vi "TrigerDelayer_ABCDEFGHDelay_Set.vi"(8 "error in (no error)":errorcluster, 10 "ABCDEFGH Delay(ns)":T1, 11 "VISA Refnum in":refnum<visa-resource-name>) -> (0 "error out":errorcluster, 3 "VISA Refnum out":refnum<visa-resource-name>)   [LabVIEW 2016, in "Trigger Delayer.lvlib"]
doc: "设置延时器的各个延时，用于同步。"
uses:
  TrigerDelayer_ABCDEFGHDelay_ctl.ctl
  Trigger Delayer.lvlib
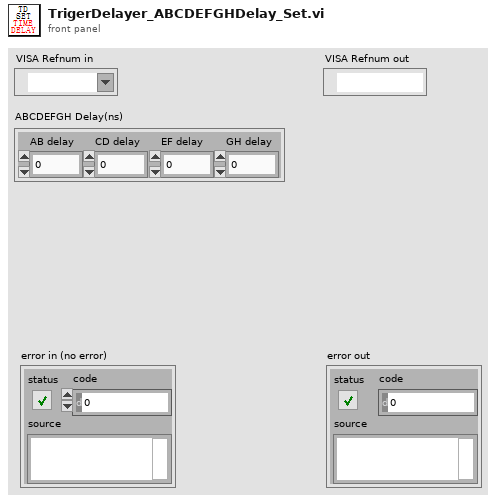
[diagram p1: front panel]
types:
  T1 = typedef "Trigger Delayer.lvlib/TrigerDelayer_ABCDEFGHDelay_ctl.ctl" = cluster{"AB delay":dbl, "CD delay":dbl, "EF delay":dbl, "GH delay":dbl}
  T2 = cluster{"AB delay":dbl, "CD delay":dbl, "EF delay":dbl, "GH delay":dbl}
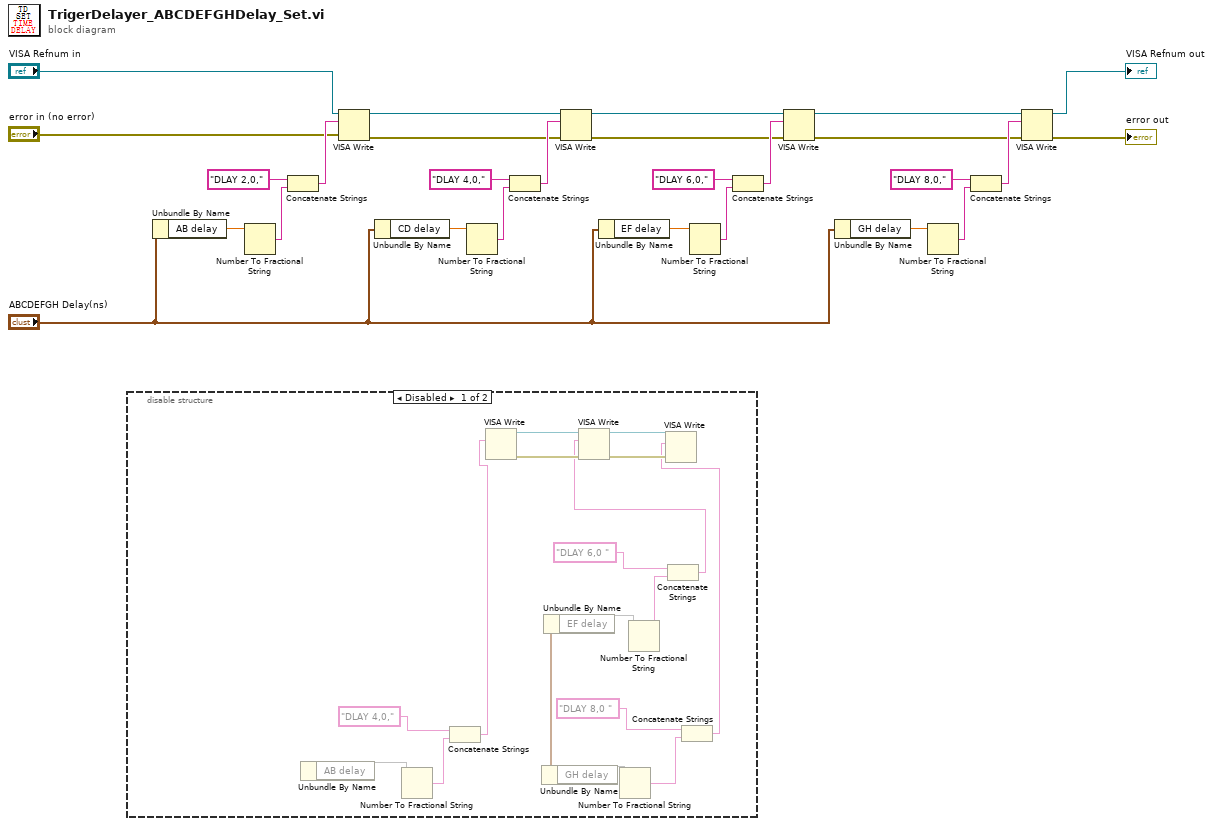
[diagram p0: block diagram]
diagram:
  n1 = disable-structure shown="Disabled" {
    frame Disabled {
      n2 = Unbundle By Name() -> (w28:T2, "AB delay"=w32)
      n3 = Number To Fractional String(number=w32) -> (F-format string=w33:string)  [unwired: 3 in]
      n4 = Concatenate Strings("DLAY 4,0,", w33) -> (w39:string)
      n5 = VISA Write(write buffer=w39) -> (VISA resource name=w42:refnum<visa-resource-name>, error in (no error)=w43:errorcluster, VISA resource name out=w44:refnum<visa-resource-name>, error out=w45:errorcluster)  [unwired: 1 out]
      n6 = Unbundle By Name() -> (w29:T2, "EF delay"=w31)
      n7 = Unbundle By Name(w29) -> ("GH delay"=w30)
      n8 = Number To Fractional String(number=w30) -> (F-format string=w38:string)  [unwired: 3 in]
      n9 = Number To Fractional String(number=w31) -> (F-format string=w35:string)  [unwired: 3 in]
      n10 = Concatenate Strings("DLAY 6,0 ", w35) -> (w40:string)
      n11 = VISA Write(VISA resource name=w44, write buffer=w40, error in (no error)=w45) -> (VISA resource name out=w46:refnum<visa-resource-name>, error out=w47:errorcluster)  [unwired: 1 out]
      n12 = Concatenate Strings("DLAY 8,0 ", w38) -> (w41:string)
      n13 = VISA Write(VISA resource name=w46, write buffer=w41, error in (no error)=w47) -> ()  [unwired: 3 out]
    }
    frame Enabled {
    }
  }
  n14 = Unbundle By Name("ABCDEFGH Delay(ns)") -> ("AB delay"=w22:dbl)
  n15 = Number To Fractional String(number=w22) -> (F-format string=w25:string)  [unwired: 3 in]
  n16 = Concatenate Strings("DLAY 2,0,", w25) -> (w27:string)
  n17 = VISA Write(VISA resource name="VISA Refnum in", write buffer=w27, error in (no error)="error in (no error)") -> (VISA resource name out=w9:refnum<visa-resource-name>, error out=w8:errorcluster)  [unwired: 1 out]
  n18 = Unbundle By Name("ABCDEFGH Delay(ns)") -> ("CD delay"=w21:dbl)
  n19 = Number To Fractional String(number=w21) -> (F-format string=w20:string)  [unwired: 3 in]
  n20 = Concatenate Strings("DLAY 4,0,", w20) -> (w18:string)
  n21 = VISA Write(VISA resource name=w9, write buffer=w18, error in (no error)=w8) -> (VISA resource name out=w7:refnum<visa-resource-name>, error out=w6:errorcluster)  [unwired: 1 out]
  n22 = Unbundle By Name("ABCDEFGH Delay(ns)") -> ("EF delay"=w14:dbl)
  n23 = Number To Fractional String(number=w14) -> (F-format string=w15:string)  [unwired: 3 in]
  n24 = Concatenate Strings("DLAY 6,0,", w15) -> (w17:string)
  n25 = VISA Write(VISA resource name=w7, write buffer=w17, error in (no error)=w6) -> (VISA resource name out=w5:refnum<visa-resource-name>, error out=w4:errorcluster)  [unwired: 1 out]
  n26 = Unbundle By Name("ABCDEFGH Delay(ns)") -> ("GH delay"=w13:dbl)
  n27 = Number To Fractional String(number=w13) -> (F-format string=w12:string)  [unwired: 3 in]
  n28 = Concatenate Strings("DLAY 8,0,", w12) -> (w10:string)
  n29 = VISA Write(VISA resource name=w5, write buffer=w10, error in (no error)=w4) -> (VISA resource name out=→"VISA Refnum out":refnum<visa-resource-name>, error out=→"error out":errorcluster)  [unwired: 1 out]
